vi "数据编码.vi"(11 "数据":dbl[](array[numeric])) -> (0 "字符串":string, 2 "16bit寄存器个数":string)   [LabVIEW 2014]
panel:
  out "32位整型":i32[](array[numeric])
  # "-9998777  分解成 C287  FFF0"
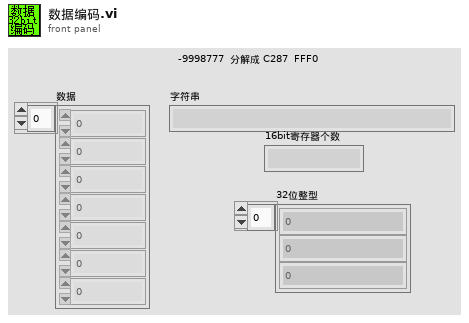
[diagram p1: front panel]
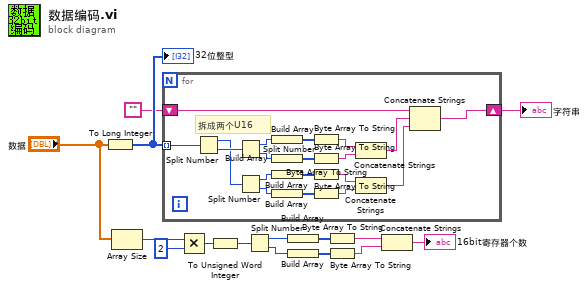
[diagram p0: block diagram]
diagram:
  n1 = To Long Integer(number="数据") -> (32bit integer=w15:i32[])
  "32位整型" <- w15
  n2 = Array Size(array="数据") -> (size(s)=w3:i32)
  n3 = for {
    tunnel: w15 -> [w26] mode=indexing
    shift-right: [w27] -> w13
    shift-left: "" -> [w28]
    # "拆成两个U16"
    n4 = Split Number(x=w26) -> (hi(x)=w18:u16, lo(x)=w25:u16)
    n5 = Split Number(x=w25) -> (hi(x)=w34:u8, lo(x)=w33:u8)
    n6 = Split Number(x=w18) -> (hi(x)=w19:u8, lo(x)=w20:u8)
    n7 = Build Array(w34) -> (w32:u8[])
    n8 = Build Array(w33) -> (w31:u8[])
    n9 = Build Array(w19) -> (w21:u8[])
    n10 = Build Array(w20) -> (w22:u8[])
    n11 = Byte Array To String(unsigned byte array=w32) -> (string=w30:string)
    n12 = Byte Array To String(unsigned byte array=w31) -> (string=w29:string)
    n13 = Byte Array To String(unsigned byte array=w21) -> (string=w23:string)
    n14 = Byte Array To String(unsigned byte array=w22) -> (string=w24:string)
    n15 = Concatenate Strings(w30, w29) -> (w17:string)
    n16 = Concatenate Strings(w23, w24) -> (w16:string)
    n17 = Concatenate Strings(w28, w17, w16) -> (w27:string)
  }
  "字符串" <- w13
  n18 = Multiply(x=w3, y=2) -> (x*y=w1:i32)
  n19 = To Unsigned Word Integer(number=w1) -> (unsigned 16bit integer=w4:u16)
  n20 = Split Number(x=w4) -> (hi(x)=w6:u8, lo(x)=w7:u8)
  n21 = Build Array(w6) -> (w8:u8[])
  n22 = Build Array(w7) -> (w9:u8[])
  n23 = Byte Array To String(unsigned byte array=w8) -> (string=w10:string)
  n24 = Byte Array To String(unsigned byte array=w9) -> (string=w11:string)
  n25 = Concatenate Strings(w10, w11) -> (→"16bit寄存器个数":string)
